vi "啮合 三角插值.vi"(8 "细分倍率":dbl=1.0, 9 "最小值":dbl, 10 "零值":dbl, 11 "最大值":dbl) -> (3 "插值结果":dbl[](array[numeric]))   [LabVIEW 2015, in "Logging.lvlib"]
uses:
  Logging.lvlib
  <vilib>/Analysis/1siggen.llb/Ramp Pattern by Samples.vi
  <vilib>/Analysis/NI_AALBase.lvlib
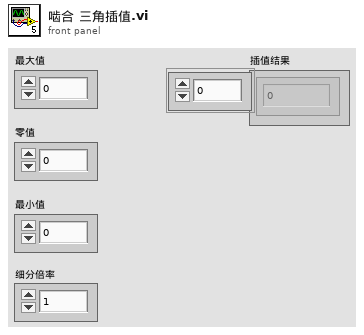
[diagram p1: front panel]
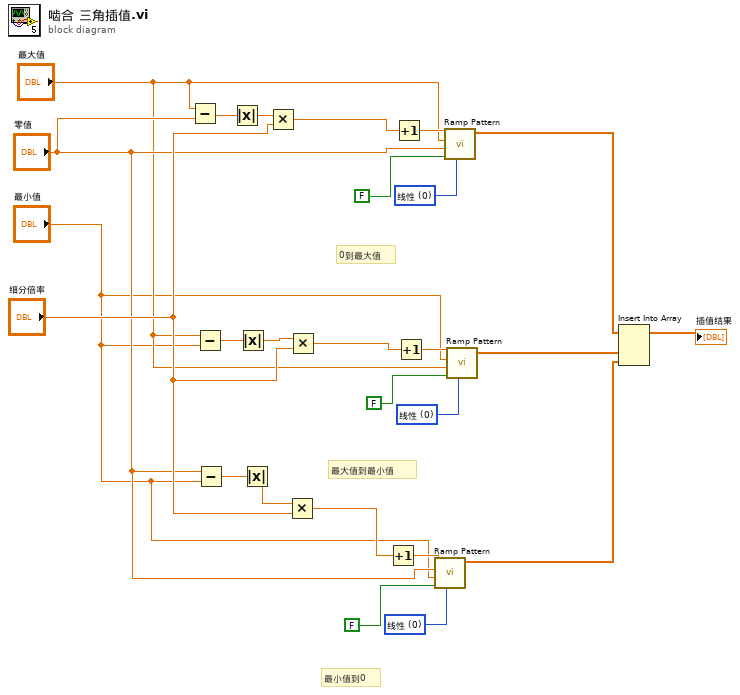
[diagram p0: block diagram]
diagram:
  w15 = u16 0 items=["线性", "对数"] ("type")
  w21 = u16 0 items=["线性", "对数"] ("type")
  w25 = u16 0 items=["线性", "对数"] ("type")
  # "最小值到0"
  # "最大值到最小值"
  # "0到最大值"
  n1 = Subtract(x="最大值", y="零值") -> (x-y=w11:dbl)
  n2 = Subtract(x="最大值", y="最小值") -> (x-y=w18:dbl)
  n3 = Subtract(x="零值", y="最小值") -> (x-y=w9:dbl)
  n4 = Absolute Value(x=w11) -> (abs(x)=w10:dbl)
  n5 = Absolute Value(x=w18) -> (abs(x)=w17:dbl)
  n6 = Absolute Value(x=w9) -> (abs(x)=w12:dbl)
  n7 = Multiply(x=w10, y="细分倍率") -> (x*y=w23:dbl)
  n8 = Multiply(x=w12, y="细分倍率") -> (x*y=w13:dbl)
  n9 = Multiply(x=w17, y="细分倍率") -> (x*y=w19:dbl)
  n10 = Increment(x=w13) -> (x+1=w14:dbl)
  n11 = Increment(x=w23) -> (x+1=w24:dbl)
  n12 = Increment(x=w19) -> (x+1=w20:dbl)
  n13 = call-poly <vilib>:"Ramp Pattern.vi"("type"=w15, "exclude end?"=FALSE, "start"="最小值", "end"="零值", "samples"=w14) -> ("Ramp Pattern"=w2:dbl[])  [unwired: 5 in, 1 out]
  n14 = call-poly <vilib>:"Ramp Pattern.vi"("type"=w25, "exclude end?"=FALSE, "start"="零值", "end"="最大值", "samples"=w24) -> ("Ramp Pattern"=w3:dbl[])  [unwired: 5 in, 1 out]
  n15 = call-poly <vilib>:"Ramp Pattern.vi"("type"=w21, "exclude end?"=FALSE, "start"="最大值", "end"="最小值", "samples"=w20) -> ("Ramp Pattern"=w6:dbl[])  [unwired: 5 in, 1 out]
  n16 = Insert Into Array(array=w3, new element #1=w6, new element #2=w2) -> (→"插值结果":dbl[])  [unwired: 1 in]
